vi "apply_scan_mode.vi"(6 "Mi (0 indexed)":i32, 9 "vector in":dbl[](array[numeric]), 10 "scan mode":T1=enum."random access") -> (1 "indices w.r.t. list":i32[](array[numeric]), 2 "vector out":dbl[](array[numeric]))   [LabVIEW 2015]
uses:
  scan_mode.ctl
  <vilib>/Analysis/1siggen.llb/Riffle Array (DBL).vi
  <vilib>/Analysis/NI_AALBase.lvlib
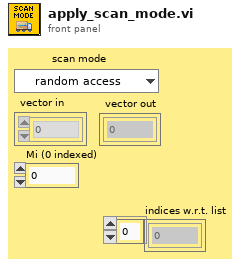
[diagram p1: front panel]
types:
  T1 = typedef "scan_mode.ctl" = enum16{"list", "reverse list", "random access", "binary riffle", "bit-flip binary riffle", "random binary riffle", "1st order TMS", "2nd order TMS", "3rd order TMS", "ad infinitum TMS", "RBR + TMS1", "RBR + TMS2", "RBR + TMS3", "RBR + TMS"}
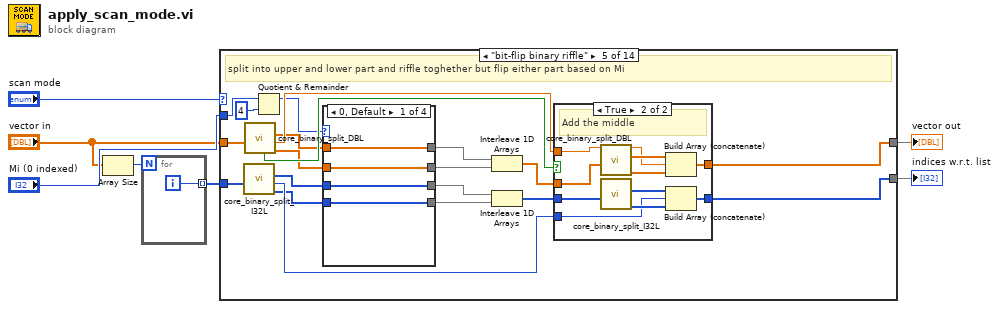
[diagram p0: block diagram]
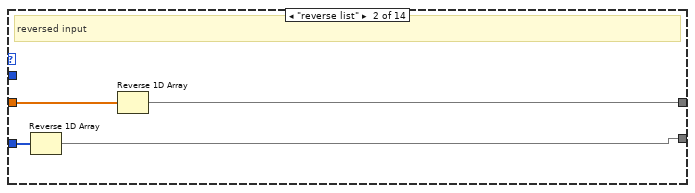
[diagram p3: hidden frame]
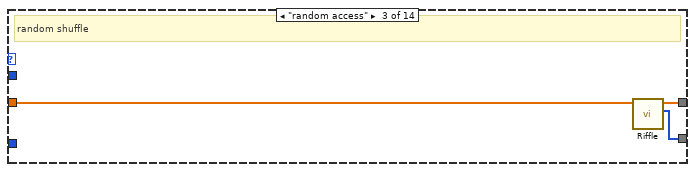
[diagram p4: hidden frame]
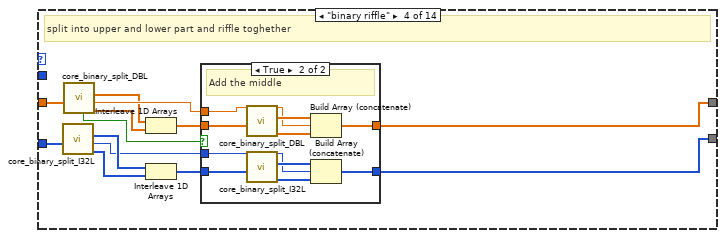
[diagram p5: hidden frame]
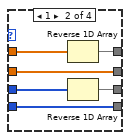
[diagram p7: hidden frame]
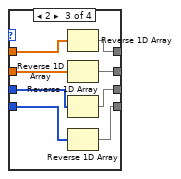
[diagram p8: hidden frame]
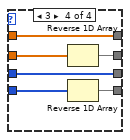
[diagram p9: hidden frame]
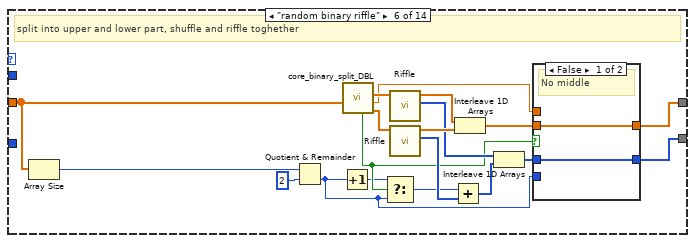
[diagram p11: hidden frame]
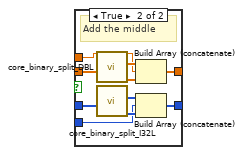
[diagram p12: hidden frame]
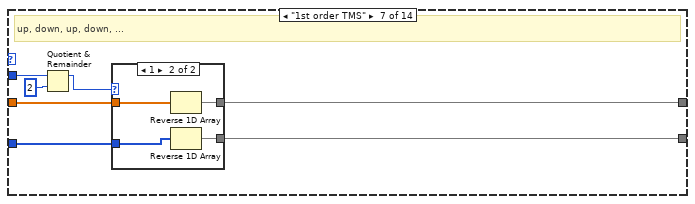
[diagram p13: hidden frame]
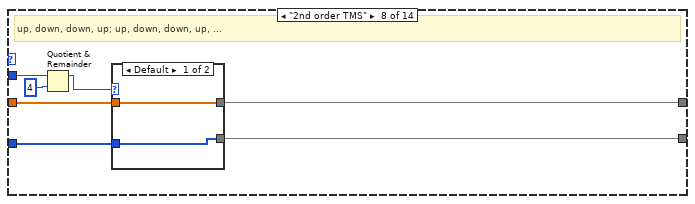
[diagram p15: hidden frame]
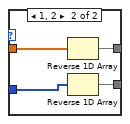
[diagram p16: hidden frame]
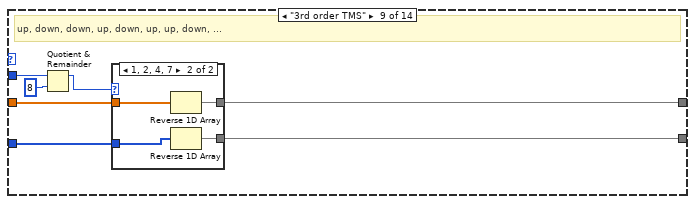
[diagram p17: hidden frame]
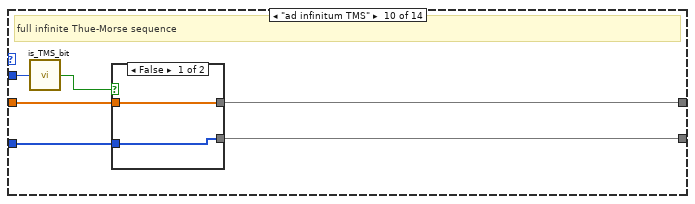
[diagram p19: hidden frame]
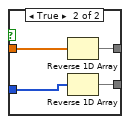
[diagram p20: hidden frame]
diagram:
  n1 = Array Size(array="vector in") -> (size(s)=w3:i32)
  n2 = for {
    N: w3 -> [_]
    tunnel: [w8] -> w1 mode=indexing
    i -> [w8]
  }
  n3 = case shown="\"bit-flip binary riffle\"" "scan mode" {
    tunnel: [w10 w13 w16 w18 w54 w110 w135 w147 w156 w174 w182 w223 w265 w308] -> w6
    tunnel: "vector in" -> [w10 w14 w17 w27 w56 w105 w136 w146 w158 w173 w188 w226 w268 w311]
    tunnel: "Mi (0 indexed)" -> [_ _ _ _ w52 _ w131 w143 w160 w170 w184 w225 w267 w310]
    tunnel: [w9 w12 w15 w19 w55 w109 w133 w145 w157 w171 w181 w224 w266 w307] -> w4
    tunnel: w1 -> [w9 w11 _ w24 w57 _ w134 w144 w159 w172 _ _ _ _]
    frame "list", Default {
      # "just like the input"
    }
    frame "reverse list" {
      # "reversed input"
      n4 = Reverse 1D Array(array=w11) -> (reversed array=w12:i32[])
      n5 = Reverse 1D Array(array=w14) -> (reversed array=w13:dbl[])
    }
    frame "random access" {
      # "random shuffle"
      n6 = call-poly <vilib>:"Riffle.vi"("X"=w17) -> ("Riffled Index"=w15:i32[], "Riffled {X}"=w16:dbl[])  [unwired: 8 in, 1 out]
    }
    frame "binary riffle" {
      # "split into upper and lower part and riffle toghether"
      n7 = call "core_binary_split_I32L.vi"("vector in"=w24) -> ("back"=w22:i32[], "middle"=w21:i32, "front"=w23:i32[])  [unwired: 7 in, 1 out]
      n8 = call "core_binary_split_DBL.vi"("vector in"=w27) -> ("back"=w25:dbl[], "middle"=w29:dbl, "front"=w26:dbl[], "odd length?"=w28:bool)  [unwired: 7 in]
      n9 = Interleave 1D Arrays(w26, w25) -> (w30:dbl[])
      n10 = Interleave 1D Arrays(w23, w22) -> (w20:i32[])
      n11 = case shown="True" w28 {
        tunnel: w30 -> [w32 w42]
        tunnel: [w32 w38] -> w18
        tunnel: [w31 w35] -> w19
        tunnel: w29 -> [_ w40]
        tunnel: w21 -> [_ w33]
        tunnel: w20 -> [w31 w34]
        frame False {
          # "No middle"
        }
        frame True {
          # "Add the middle"
          n12 = call "core_binary_split_DBL.vi"("vector in"=w42) -> ("back"=w39:dbl[], "front"=w41:dbl[])  [unwired: 7 in, 2 out]
          n13 = call "core_binary_split_I32L.vi"("vector in"=w34) -> ("back"=w36:i32[], "front"=w37:i32[])  [unwired: 7 in, 2 out]
          n14 = Build Array (concatenate)(w41, w40, w39) -> (w38:dbl[])
          n15 = Build Array (concatenate)(w37, w33, w36) -> (w35:i32[])
        }
      }
    }
    frame "bit-flip binary riffle" {
      # "split into upper and lower part and riffle toghether but flip either part based on Mi"
      n16 = call "core_binary_split_I32L.vi"("vector in"=w57) -> ("back"=w46:i32[], "middle"=w59:i32, "front"=w50:i32[])  [unwired: 7 in, 1 out]
      n17 = call "core_binary_split_DBL.vi"("vector in"=w56) -> ("back"=w44:dbl[], "middle"=w61:dbl, "front"=w48:dbl[], "odd length?"=w60:bool)  [unwired: 7 in]
      n18 = Quotient & Remainder(x=w52, y=4) -> (x-y*floor(x/y)=w51:i32)  [unwired: 1 out]
      n19 = case shown="0, Default" w51 {
        tunnel: w50 -> [w66 w72 w80 w84]
        tunnel: [w66 w71 w79 w84] -> w49
        tunnel: w48 -> [w65 w70 w78 w81]
        tunnel: [w65 w69 w77 w81] -> w47
        tunnel: w46 -> [w64 w68 w76 w86]
        tunnel: [w64 w68 w75 w85] -> w45
        tunnel: w44 -> [w63 w67 w74 w83]
        tunnel: [w63 w67 w73 w82] -> w43
        frame 0, Default {
        }
        frame 1 {
          n20 = Reverse 1D Array(array=w70) -> (reversed array=w69:dbl[])
          n21 = Reverse 1D Array(array=w72) -> (reversed array=w71:i32[])
        }
        frame 2 {
          n22 = Reverse 1D Array(array=w78) -> (reversed array=w77:dbl[])
          n23 = Reverse 1D Array(array=w74) -> (reversed array=w73:dbl[])
          n24 = Reverse 1D Array(array=w80) -> (reversed array=w79:i32[])
          n25 = Reverse 1D Array(array=w76) -> (reversed array=w75:i32[])
        }
        frame 3 {
          n26 = Reverse 1D Array(array=w83) -> (reversed array=w82:dbl[])
          n27 = Reverse 1D Array(array=w86) -> (reversed array=w85:i32[])
        }
      }
      n28 = Interleave 1D Arrays(w47, w43) -> (w62:dbl[])
      n29 = Interleave 1D Arrays(w49, w45) -> (w58:i32[])
      n30 = case shown="True" w60 {
        tunnel: w62 -> [w88 w98]
        tunnel: [w88 w94] -> w54
        tunnel: [w87 w91] -> w55
        tunnel: w61 -> [_ w96]
        tunnel: w59 -> [_ w89]
        tunnel: w58 -> [w87 w90]
        frame False {
          # "No middle"
        }
        frame True {
          # "Add the middle"
          n31 = call "core_binary_split_DBL.vi"("vector in"=w98) -> ("back"=w95:dbl[], "front"=w97:dbl[])  [unwired: 7 in, 2 out]
          n32 = call "core_binary_split_I32L.vi"("vector in"=w90) -> ("back"=w92:i32[], "front"=w93:i32[])  [unwired: 7 in, 2 out]
          n33 = Build Array (concatenate)(w97, w96, w95) -> (w94:dbl[])
          n34 = Build Array (concatenate)(w93, w89, w92) -> (w91:i32[])
        }
      }
    }
    frame "random binary riffle" {
      # "split into upper and lower part, shuffle and riffle toghether"
      n35 = Array Size(array=w105) -> (size(s)=w107:i32)
      n36 = Quotient & Remainder(x=w107, y=2) -> (floor(x/y)=w99:i32)  [unwired: 1 out]
      n37 = Increment(x=w99) -> (x+1=w101:i32)
      n38 = call "core_binary_split_DBL.vi"("vector in"=w105) -> ("back"=w116:dbl[], "middle"=w108:dbl, "front"=w117:dbl[], "odd length?"=w102:bool)  [unwired: 7 in]
      n39 = Select(t=w101, s=w102, f=w99) -> (s? t:f=w100:i32)
      n40 = call-poly <vilib>:"Riffle.vi"("X"=w117) -> ("Riffled Index"=w113:i32[], "Riffled {X}"=w115:dbl[])  [unwired: 8 in, 1 out]
      n41 = call-poly <vilib>:"Riffle.vi"("X"=w116) -> ("Riffled Index"=w104:i32[], "Riffled {X}"=w114:dbl[])  [unwired: 8 in, 1 out]
      n42 = Add(x=w100, y=w104) -> (x+y=w103:i32[])
      n43 = Interleave 1D Arrays(w115, w114) -> (w112:dbl[])
      n44 = Interleave 1D Arrays(w113, w103) -> (w111:i32[])
      n45 = case shown="False" w102 {
        tunnel: w112 -> [w119 w129]
        tunnel: w111 -> [w118 w128]
        tunnel: [w119 w124] -> w110
        tunnel: [w118 w120] -> w109
        tunnel: w108 -> [_ w126]
        tunnel: w99 -> [_ w121]
        frame False {
          # "No middle"
        }
        frame True {
          # "Add the middle"
          n46 = call "core_binary_split_DBL.vi"("vector in"=w129) -> ("back"=w125:dbl[], "front"=w127:dbl[])  [unwired: 7 in, 2 out]
          n47 = call "core_binary_split_I32L.vi"("vector in"=w128) -> ("back"=w122:i32[], "front"=w123:i32[])  [unwired: 7 in, 2 out]
          n48 = Build Array (concatenate)(w127, w126, w125) -> (w124:dbl[])
          n49 = Build Array (concatenate)(w123, w121, w122) -> (w120:i32[])
        }
      }
    }
    frame "1st order TMS" {
      # "up, down, up, down, ..."
      n50 = Quotient & Remainder(x=w131, y=2) -> (x-y*floor(x/y)=w130:i32)  [unwired: 1 out]
      n51 = case shown="1" w130 {
        tunnel: w136 -> [w138 w142]
        tunnel: [w138 w141] -> w135
        tunnel: w134 -> [w137 w140]
        tunnel: [w137 w139] -> w133
        frame 0, Default {
        }
        frame 1 {
          n52 = Reverse 1D Array(array=w142) -> (reversed array=w141:dbl[])
          n53 = Reverse 1D Array(array=w140) -> (reversed array=w139:i32[])
        }
      }
    }
    frame "2nd order TMS" {
      # "up, down, down, up; up, down, down, up, ..."
      n54 = Quotient & Remainder(x=w143, y=4) -> (x-y*floor(x/y)=w148:i32)  [unwired: 1 out]
      n55 = case shown="Default" w148 {
        tunnel: [w151 w154] -> w147
        tunnel: w146 -> [w151 w155]
        tunnel: [w150 w152] -> w145
        tunnel: w144 -> [w150 w153]
        frame Default {
        }
        frame 1, 2 {
          n56 = Reverse 1D Array(array=w155) -> (reversed array=w154:dbl[])
          n57 = Reverse 1D Array(array=w153) -> (reversed array=w152:i32[])
        }
      }
    }
    frame "3rd order TMS" {
      # "up, down, down, up, down, up, up, down, ..."
      n58 = Quotient & Remainder(x=w160, y=8) -> (x-y*floor(x/y)=w161:i32)  [unwired: 1 out]
      n59 = case shown="1, 2, 4, 7" w161 {
        tunnel: [w164 w167] -> w156
        tunnel: w158 -> [w164 w168]
        tunnel: [w163 w165] -> w157
        tunnel: w159 -> [w163 w166]
        frame Default {
        }
        frame 1, 2, 4, 7 {
          n60 = Reverse 1D Array(array=w168) -> (reversed array=w167:dbl[])
          n61 = Reverse 1D Array(array=w166) -> (reversed array=w165:i32[])
        }
      }
    }
    frame "ad infinitum TMS" {
      # "full infinite Thue-Morse sequence"
      n62 = call "is_TMS_bit.vi"("Mi (0 indexed)"=w170) -> ("TMS bit"=w169:bool)  [unwired: 8 in]
      n63 = case shown="False" w169 {
        tunnel: [w176 w179] -> w174
        tunnel: w173 -> [w176 w180]
        tunnel: w172 -> [w175 w178]
        tunnel: [w175 w177] -> w171
        frame False {
        }
        frame True {
          n64 = Reverse 1D Array(array=w180) -> (reversed array=w179:dbl[])
          n65 = Reverse 1D Array(array=w178) -> (reversed array=w177:i32[])
        }
      }
    }
    frame "RBR + TMS1" {
      # "Randomised binary riffle + 1st order Thue-Morse"
      n66 = Array Size(array=w188) -> (size(s)=w196:i32)
      n67 = Quotient & Remainder(x=w196, y=2) -> (floor(x/y)=w189:i32)  [unwired: 1 out]
      n68 = Increment(x=w189) -> (x+1=w191:i32)
      n69 = call "core_binary_split_DBL.vi"("vector in"=w188) -> ("back"=w203:dbl[], "middle"=w197:dbl, "front"=w204:dbl[], "odd length?"=w192:bool)  [unwired: 7 in]
      n70 = Select(t=w191, s=w192, f=w189) -> (s? t:f=w190:i32)
      n71 = call-poly <vilib>:"Riffle.vi"("X"=w204) -> ("Riffled Index"=w200:i32[], "Riffled {X}"=w202:dbl[])  [unwired: 8 in, 1 out]
      n72 = call-poly <vilib>:"Riffle.vi"("X"=w203) -> ("Riffled Index"=w194:i32[], "Riffled {X}"=w201:dbl[])  [unwired: 8 in, 1 out]
      n73 = Interleave 1D Arrays(w202, w201) -> (w199:dbl[])
      n74 = Add(x=w190, y=w194) -> (x+y=w193:i32[])
      n75 = Interleave 1D Arrays(w200, w193) -> (w198:i32[])
      n76 = case shown="False" w192 {
        tunnel: w199 -> [w212 w222]
        tunnel: w198 -> [w211 w221]
        tunnel: [w212 w217] -> w187
        tunnel: [w211 w213] -> w186
        tunnel: w197 -> [_ w219]
        tunnel: w189 -> [_ w214]
        frame False {
          # "No middle"
        }
        frame True {
          # "Add the middle"
          n77 = call "core_binary_split_DBL.vi"("vector in"=w222) -> ("back"=w218:dbl[], "front"=w220:dbl[])  [unwired: 7 in, 2 out]
          n78 = call "core_binary_split_I32L.vi"("vector in"=w221) -> ("back"=w215:i32[], "front"=w216:i32[])  [unwired: 7 in, 2 out]
          n79 = Build Array (concatenate)(w220, w219, w218) -> (w217:dbl[])
          n80 = Build Array (concatenate)(w216, w214, w215) -> (w213:i32[])
        }
      }
      n81 = Quotient & Remainder(x=w184, y=2) -> (x-y*floor(x/y)=w183:i32)  [unwired: 1 out]
      n82 = case shown="Default" w183 {
        tunnel: w187 -> [w206 w210]
        tunnel: [w206 w209] -> w182
        tunnel: w186 -> [w205 w208]
        tunnel: [w205 w207] -> w181
        frame Default {
        }
        frame 1 {
          n83 = Reverse 1D Array(array=w210) -> (reversed array=w209:dbl[])
          n84 = Reverse 1D Array(array=w208) -> (reversed array=w207:i32[])
        }
      }
    }
    frame "RBR + TMS2" {
      # "Randomised binary riffle + 2st order Thue-Morse"
      n85 = Array Size(array=w226) -> (size(s)=w238:i32)
      n86 = Quotient & Remainder(x=w238, y=2) -> (floor(x/y)=w231:i32)  [unwired: 1 out]
      n87 = Increment(x=w231) -> (x+1=w233:i32)
      n88 = call "core_binary_split_DBL.vi"("vector in"=w226) -> ("back"=w245:dbl[], "middle"=w239:dbl, "front"=w246:dbl[], "odd length?"=w234:bool)  [unwired: 7 in]
      n89 = Select(t=w233, s=w234, f=w231) -> (s? t:f=w232:i32)
      n90 = call-poly <vilib>:"Riffle.vi"("X"=w246) -> ("Riffled Index"=w242:i32[], "Riffled {X}"=w244:dbl[])  [unwired: 8 in, 1 out]
      n91 = call-poly <vilib>:"Riffle.vi"("X"=w245) -> ("Riffled Index"=w236:i32[], "Riffled {X}"=w243:dbl[])  [unwired: 8 in, 1 out]
      n92 = Interleave 1D Arrays(w244, w243) -> (w241:dbl[])
      n93 = Add(x=w232, y=w236) -> (x+y=w235:i32[])
      n94 = Interleave 1D Arrays(w242, w235) -> (w240:i32[])
      n95 = case shown="False" w234 {
        tunnel: w241 -> [w254 w264]
        tunnel: w240 -> [w253 w263]
        tunnel: [w254 w259] -> w230
        tunnel: [w253 w255] -> w229
        tunnel: w239 -> [_ w261]
        tunnel: w231 -> [_ w256]
        frame False {
          # "No middle"
        }
        frame True {
          # "Add the middle"
          n96 = call "core_binary_split_DBL.vi"("vector in"=w264) -> ("back"=w260:dbl[], "front"=w262:dbl[])  [unwired: 7 in, 2 out]
          n97 = call "core_binary_split_I32L.vi"("vector in"=w263) -> ("back"=w257:i32[], "front"=w258:i32[])  [unwired: 7 in, 2 out]
          n98 = Build Array (concatenate)(w262, w261, w260) -> (w259:dbl[])
          n99 = Build Array (concatenate)(w258, w256, w257) -> (w255:i32[])
        }
      }
      n100 = Quotient & Remainder(x=w225, y=4) -> (x-y*floor(x/y)=w227:i32)  [unwired: 1 out]
      n101 = case shown="1, 2" w227 {
        tunnel: w230 -> [w248 w252]
        tunnel: [w248 w251] -> w223
        tunnel: w229 -> [w247 w250]
        tunnel: [w247 w249] -> w224
        frame Default {
        }
        frame 1, 2 {
          n102 = Reverse 1D Array(array=w252) -> (reversed array=w251:dbl[])
          n103 = Reverse 1D Array(array=w250) -> (reversed array=w249:i32[])
        }
      }
    }
    frame "RBR + TMS3" {
      # "Randomised binary riffle + 3rd order Thue-Morse"
      n104 = Array Size(array=w268) -> (size(s)=w280:i32)
      n105 = Quotient & Remainder(x=w280, y=2) -> (floor(x/y)=w273:i32)  [unwired: 1 out]
      n106 = Increment(x=w273) -> (x+1=w275:i32)
      n107 = call "core_binary_split_DBL.vi"("vector in"=w268) -> ("back"=w287:dbl[], "middle"=w281:dbl, "front"=w288:dbl[], "odd length?"=w276:bool)  [unwired: 7 in]
      n108 = Select(t=w275, s=w276, f=w273) -> (s? t:f=w274:i32)
      n109 = call-poly <vilib>:"Riffle.vi"("X"=w288) -> ("Riffled Index"=w284:i32[], "Riffled {X}"=w286:dbl[])  [unwired: 8 in, 1 out]
      n110 = call-poly <vilib>:"Riffle.vi"("X"=w287) -> ("Riffled Index"=w278:i32[], "Riffled {X}"=w285:dbl[])  [unwired: 8 in, 1 out]
      n111 = Interleave 1D Arrays(w286, w285) -> (w283:dbl[])
      n112 = Add(x=w274, y=w278) -> (x+y=w277:i32[])
      n113 = Interleave 1D Arrays(w284, w277) -> (w282:i32[])
      n114 = case shown="False" w276 {
        tunnel: w283 -> [w296 w306]
        tunnel: w282 -> [w295 w305]
        tunnel: [w296 w301] -> w272
        tunnel: [w295 w297] -> w271
        tunnel: w281 -> [_ w303]
        tunnel: w273 -> [_ w298]
        frame False {
          # "No middle"
        }
        frame True {
          # "Add the middle"
          n115 = call "core_binary_split_DBL.vi"("vector in"=w306) -> ("back"=w302:dbl[], "front"=w304:dbl[])  [unwired: 7 in, 2 out]
          n116 = call "core_binary_split_I32L.vi"("vector in"=w305) -> ("back"=w299:i32[], "front"=w300:i32[])  [unwired: 7 in, 2 out]
          n117 = Build Array (concatenate)(w304, w303, w302) -> (w301:dbl[])
          n118 = Build Array (concatenate)(w300, w298, w299) -> (w297:i32[])
        }
      }
      n119 = Quotient & Remainder(x=w267, y=8) -> (x-y*floor(x/y)=w269:i32)  [unwired: 1 out]
      n120 = case shown="1, 2, 4, 7" w269 {
        tunnel: w272 -> [w290 w294]
        tunnel: [w290 w293] -> w265
        tunnel: w271 -> [w289 w292]
        tunnel: [w289 w291] -> w266
        frame Default {
        }
        frame 1, 2, 4, 7 {
          n121 = Reverse 1D Array(array=w294) -> (reversed array=w293:dbl[])
          n122 = Reverse 1D Array(array=w292) -> (reversed array=w291:i32[])
        }
      }
    }
    frame "RBR + TMS" {
      # "Randomised binary riffle + Thue-Morse sequencing"
      n123 = Array Size(array=w311) -> (size(s)=w321:i32)
      n124 = Quotient & Remainder(x=w321, y=2) -> (floor(x/y)=w314:i32)  [unwired: 1 out]
      n125 = Increment(x=w314) -> (x+1=w316:i32)
      n126 = call "core_binary_split_DBL.vi"("vector in"=w311) -> ("back"=w328:dbl[], "middle"=w322:dbl, "front"=w329:dbl[], "odd length?"=w317:bool)  [unwired: 7 in]
      n127 = Select(t=w316, s=w317, f=w314) -> (s? t:f=w315:i32)
      n128 = call-poly <vilib>:"Riffle.vi"("X"=w329) -> ("Riffled Index"=w325:i32[], "Riffled {X}"=w327:dbl[])  [unwired: 8 in, 1 out]
      n129 = call-poly <vilib>:"Riffle.vi"("X"=w328) -> ("Riffled Index"=w319:i32[], "Riffled {X}"=w326:dbl[])  [unwired: 8 in, 1 out]
      n130 = Interleave 1D Arrays(w327, w326) -> (w324:dbl[])
      n131 = Add(x=w315, y=w319) -> (x+y=w318:i32[])
      n132 = Interleave 1D Arrays(w325, w318) -> (w323:i32[])
      n133 = case shown="False" w317 {
        tunnel: w324 -> [w337 w347]
        tunnel: w323 -> [w336 w346]
        tunnel: [w337 w342] -> w313
        tunnel: [w336 w338] -> w312
        tunnel: w322 -> [_ w344]
        tunnel: w314 -> [_ w339]
        frame False {
          # "No middle"
        }
        frame True {
          # "Add the middle"
          n134 = call "core_binary_split_DBL.vi"("vector in"=w347) -> ("back"=w343:dbl[], "front"=w345:dbl[])  [unwired: 7 in, 2 out]
          n135 = call "core_binary_split_I32L.vi"("vector in"=w346) -> ("back"=w340:i32[], "front"=w341:i32[])  [unwired: 7 in, 2 out]
          n136 = Build Array (concatenate)(w345, w344, w343) -> (w342:dbl[])
          n137 = Build Array (concatenate)(w341, w339, w340) -> (w338:i32[])
        }
      }
      n138 = call "is_TMS_bit.vi"("Mi (0 indexed)"=w310) -> ("TMS bit"=w309:bool)  [unwired: 8 in]
      n139 = case shown="False" w309 {
        tunnel: w313 -> [w331 w335]
        tunnel: [w331 w334] -> w308
        tunnel: w312 -> [w330 w333]
        tunnel: [w330 w332] -> w307
        frame False {
        }
        frame True {
          n140 = Reverse 1D Array(array=w335) -> (reversed array=w334:dbl[])
          n141 = Reverse 1D Array(array=w333) -> (reversed array=w332:i32[])
        }
      }
    }
  }
  "vector out" <- w6
  "indices w.r.t. list" <- w4
